vi "ExOpenCamGlobal.vi"() -> ()   [LabVIEW 2010]
uses:
  GlbCamHndls.vi
panel:
  out "error out":errorcluster
  in  "error in (no error)":errorcluster
  in  "Number of Cameras":u32=1 min=1 step=1
  # "ExOpenCamGlobal.vi : this vi opens n cameras\nfor the global camera example. It stores them\nin a global camera handle array."
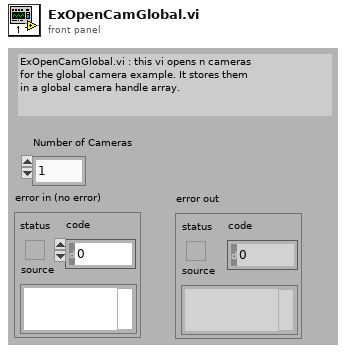
[diagram p1: front panel]
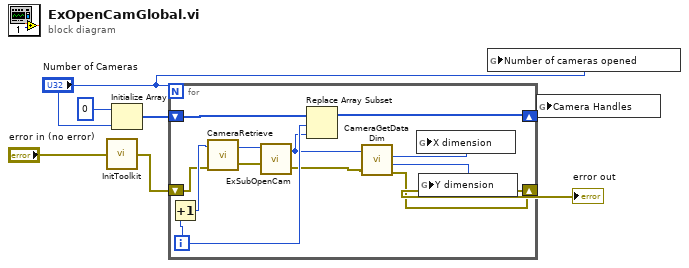
[diagram p0: block diagram]
diagram:
  n1 = call <userlib>:"InitToolkit.vi"("error in"="error in (no error)") -> ("error out"=w5:errorcluster)
  n2 = Initialize Array(0, "Number of Cameras") -> (w7:i32[])
  n3 = for {
    N: "Number of Cameras" -> [_]
    shift-right: [w14] -> w2
    shift-left: w7 -> [w16]
    shift-right: [w8] -> w3
    shift-left: w5 -> [w17]
    i -> [w19]
    n4 = Increment(x=w19) -> (x+1=w18:i32)
    n5 = call <userlib>:"CameraRetrieve.vi"("error in"=w17, "Camera Index"=w18) -> ("error out"=w12:errorcluster, "Device ID"=w15:u32)
    n6 = call "ExSubOpenCam.vi"("error in (no error)"=w12, "Camera Device ID"=w15) -> ("error out"=w11:errorcluster, "Camera Handle"=w13:u32)
    n7 = Replace Array Subset(array=w16, new element=w13, index=w19) -> (w14:i32[])
    n8 = call <userlib>:"CameraGetDataDim.vi"("Camera Handle"=w13, "error in"=w11) -> ("Xdim"=w10:u32, "Ydim"=w9:u32, "error out"=w8:errorcluster)  [unwired: 1 out]
    n9 = global write "GlbCamHndls.vi" "X dimension"(w10) -> ()
    n10 = global write "GlbCamHndls.vi" "Y dimension"(w9) -> ()
  }
  "error out" <- w3
  n11 = global write "GlbCamHndls.vi" "Number of cameras opened"("Number of Cameras") -> ()
  n12 = global write "GlbCamHndls.vi" "Camera Handles"(w2) -> ()
